vi "Teardown.vi"(8 "Error In":errorcluster, 10 "Known Host":refnum<class "KnownHost.lvclass">, 11 "Known Hosts":refnum<class "KnownHosts.lvclass">) -> (0 "Error Out":errorcluster)   [LabVIEW 2018, in "Tests.lvlib" / "KnownHost.lvlib"]
uses:
  KnownHost.lvlib
  src/Toolkit/API/KnownHost/KnownHost.lvclass
  src/Toolkit/API/KnownHosts/KnownHosts.lvclass
  src/Toolkit/API/Session/Session.lvclass
  src/Toolkit/API/SSH/SSH.lvclass
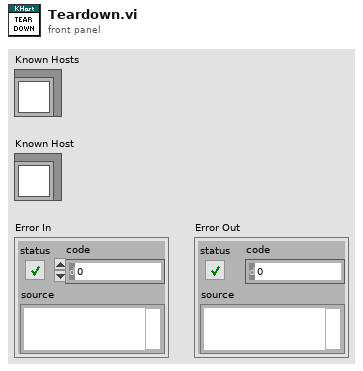
[diagram p1: front panel]
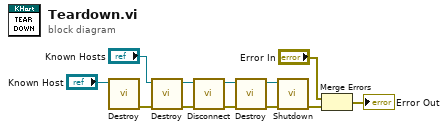
[diagram p0: block diagram]
diagram:
  n1 = call "Destroy.vi"("Known Host"="Known Host") -> ("Error Out"=w5:errorcluster)  [unwired: 9 in, 1 out]
  n2 = call "Destroy.vi"("Error In"=w5, "KnownHosts"="Known Hosts") -> ("Error Out"=w4:errorcluster, "Session"=w1:refnum<class "Session.lvclass">)  [unwired: 8 in]
  n3 = call "Disconnect.vi"("Error In"=w4, "Session In"=w1) -> ("Error Out"=w12:errorcluster, "Sesssion Out"=w11:refnum<class "Session.lvclass">)  [unwired: 8 in]
  n4 = call "Destroy.vi"("Error In"=w12, "Session"=w11) -> ("Error Out"=w9:errorcluster, "SSH"=w8:refnum<class "SSH.lvclass">)  [unwired: 8 in]
  n5 = call "Shutdown.vi"("Error In"=w9, "SSH"=w8) -> ("Error Out"=w10:errorcluster)  [unwired: 9 in]
  n6 = Merge Errors("Error In", w10) -> (→"Error Out":errorcluster)
